vi "Read Key List.vi"(8 "error in":errorcluster, 11 "Device in":refnum<class>) -> (0 "error out":errorcluster, 2 "Required Keys":string[](array[string]), 3 "Device out":refnum<class>)   [LabVIEW 2019]
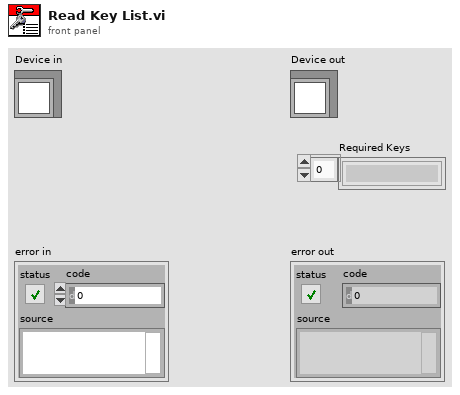
[diagram p1: front panel]
types:
  T1 = enum32{"invalid scope", "public", "private", "protected", "community"}
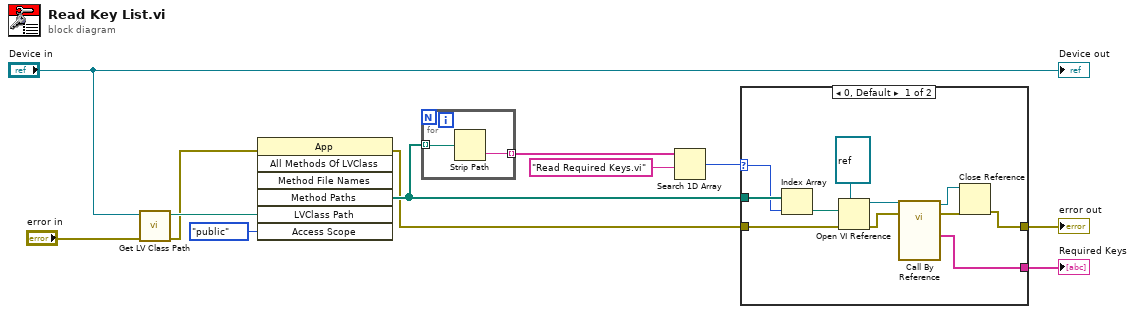
[diagram p0: block diagram]
diagram:
  n1 = call <vilib>:"Get LV Class Path.vi"("error in (no error)"="error in", "object"="Device in") -> ("error out"=w8:errorcluster, "class path"=w11:path)  [unwired: 8 in]
  n2 = invoke class="App" method="All Methods Of LVClass"(error in=w8, "LVClass Path"=w11, "Access Scope"=T1."public") -> (error out=w3:errorcluster, "Method Paths"=w4:path[])  [unwired: 4 in, 5 out]
  n3 = for {
    tunnel: w4 -> [w14] mode=indexing
    tunnel: [w13] -> w7 mode=indexing
    n4 = Strip Path(path=w14) -> (name=w13:string)  [unwired: 1 out]
  }
  n5 = Search 1D Array(1D array=w7, element="Read Required Keys.vi" ("string")) -> (index of element=w5:i32)  [unwired: 1 in]
  n6 = case shown="0, Default" w5 {
    selector: w5 -> [w24 _]
    tunnel: w4 -> [w25 _]
    tunnel: w3 -> [w17 w26]
    tunnel: [w16 w26] -> w2
    tunnel: [w15 _] -> w1
    frame 0, Default {
      n7 = Index Array(array=w25, index=w24) -> (element=w23:path)
      n8 = Open VI Reference(type specifier VI Refnum (for type only)=refnum<vi> refnum, vi path=w23, error in (no error)=w17) -> (vi reference=w21:refnum<vi>, error out=w20:errorcluster)  [unwired: 3 in]
      n9 = call-by-ref "?"(reference=w21, error in=w20) -> (reference out=w18:refnum<vi>, error out=w19:errorcluster, "Required Keys"=w15:string[])  [unwired: 11 in]
      n10 = Close Reference(reference=w18, error in (no error)=w19) -> (error out=w16:errorcluster)
    }
    frame -1 {
    }
  }
  "error out" <- w2
  "Required Keys" <- w1
  "Device out" <- "Device in"
